vi "Main.vi"() -> ()   [LabVIEW 2019]
uses:
  Classes/House.lvclass
  Classes/Shower.lvclass
  C:/Users/crawler/Documents/LabVIEW/Robertian_HousesCalc/Classes/Furniture.lvclass
  Classes/RoomB.lvclass
  C:/Users/crawler/Documents/LabVIEW/Robertian_HousesCalc/Classes/Room.lvclass
  Classes/Couch.lvclass
  Classes/TV.lvclass
  Classes/RoomA.lvclass
  Classes/Bed.lvclass
  Classes/RoomC.lvclass
  Classes/Room.lvclass
  Classes/Furniture.lvclass
panel:
  out "sum":dbl
  out "House out":refnum<class "House.lvclass">
  in  "Shower":i32=3
  in  "Livingroom":i32=3
  in  "Bedroom":i32
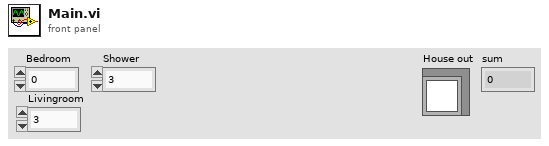
[diagram p1: front panel]
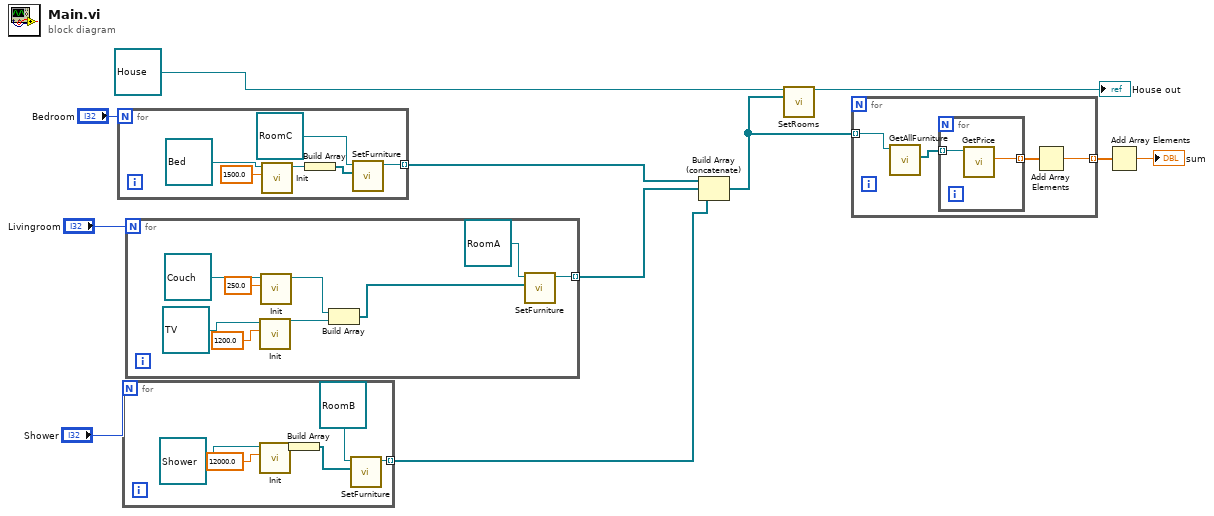
[diagram p0: block diagram]
diagram:
  n1 = for {
    N: "Bedroom" -> [_]
    tunnel: [w13] -> w7 mode=indexing
    n2 = call-dynamic "Init.vi"("Price"=1500.0, "Bed in"=refnum<class "Bed.lvclass"> refnum ("Bed.lvclass")) -> ("Bed out"=w14:refnum<class "Bed.lvclass">)  [unwired: 8 in, 1 out]
    n3 = Build Array(w14) -> (w12:refnum<class "Bed.lvclass">[])
    n4 = call-dynamic "SetFurniture.vi"("Furniture"=w12, "RoomC in"=refnum<class "RoomC.lvclass"> refnum ("RoomC.lvclass")) -> ("RoomC out"=w13:refnum<class "RoomC.lvclass">)  [unwired: 8 in, 1 out]
  }
  n5 = for {
    N: "Shower" -> [_]
    tunnel: [w19] -> w5 mode=indexing
    n6 = call-dynamic "Init.vi"("Price"=12000.0, "Shower in"=refnum<class "Shower.lvclass"> refnum ("Shower.lvclass")) -> ("Shower out"=w21:refnum<class "Shower.lvclass">)  [unwired: 8 in, 1 out]
    n7 = Build Array(w21) -> (w18:refnum<class "Shower.lvclass">[])
    n8 = call-dynamic "SetFurniture.vi"("Furniture"=w18, "RoomB in"=refnum<class "RoomB.lvclass"> refnum ("RoomB.lvclass")) -> ("RoomB out"=w19:refnum<class "RoomB.lvclass">)  [unwired: 8 in, 1 out]
  }
  n9 = for {
    N: "Livingroom" -> [_]
    tunnel: [w24] -> w6 mode=indexing
    n10 = call-dynamic "Init.vi"("Price"=1200.0, "TV in"=refnum<class "TV.lvclass"> refnum ("TV.lvclass")) -> ("TV out"=w27:refnum<class "TV.lvclass">)  [unwired: 8 in, 1 out]
    n11 = call-dynamic "Init.vi"("Price"=250.0, "Couch in"=refnum<class "Couch.lvclass"> refnum ("Couch.lvclass")) -> ("Couch out"=w28:refnum<class "Couch.lvclass">)  [unwired: 8 in, 1 out]
    n12 = Build Array(w28, w27) -> (w26:refnum<class "Furniture.lvclass">[])
    n13 = call-dynamic "SetFurniture.vi"("Furniture"=w26, "RoomA in"=refnum<class "RoomA.lvclass"> refnum ("RoomA.lvclass")) -> ("RoomA out"=w24:refnum<class "RoomA.lvclass">)  [unwired: 8 in, 1 out]
  }
  n14 = Build Array (concatenate)(w7, w6, w5) -> (w3:refnum<class "Room.lvclass">[])
  n15 = call "SetRooms.vi"("House in"=refnum<class "House.lvclass"> refnum ("House.lvclass"), "Rooms"=w3) -> ("House out"=→"House out":refnum<class "House.lvclass">)  [unwired: 12 in, 1 out]
  n16 = for {
    tunnel: w3 -> [w36] mode=indexing
    tunnel: [w33] -> w2 mode=indexing
    n17 = call-dynamic "GetAllFurniture.vi"("Room in"=w36) -> ("Furniture"=w35:refnum<class "Furniture.lvclass">[])  [unwired: 8 in, 2 out]
    n18 = for {
      tunnel: w35 -> [w38] mode=indexing
      tunnel: [w37] -> w34 mode=indexing
      n19 = call-dynamic "GetPrice.vi"("Furniture in"=w38) -> ("Price"=w37:dbl)  [unwired: 8 in, 2 out]
    }
    n20 = Add Array Elements(numeric array=w34) -> (sum=w33:dbl)
  }
  n21 = Add Array Elements(numeric array=w2) -> (sum=→"sum":dbl)
